vi "IPI_DrawLine.vi"(7 "Roi":dbl[](array[numeric]), 8 "error in (no error)":errorcluster, 9 "Distance Piex":string, 10 "Start Point":cluster{"X":dbl, "Y":dbl}, 11 "Image In":T1(plugin-control)) -> (0 "error out (no error)":errorcluster, 3 "Image Out":T1(plugin-control))   [LabVIEW 2015]
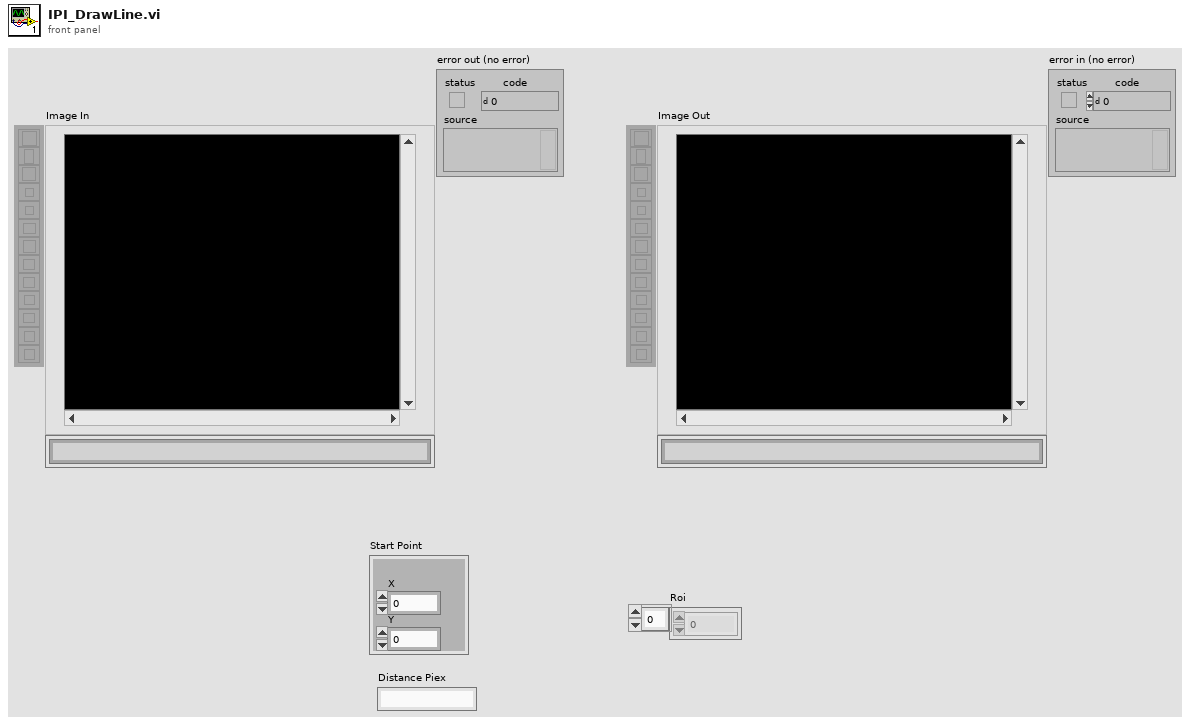
[diagram p1: front panel]
types:
  T1 = typedef "IMAQ Image.ctl" = refnum<image>
  T2 = cluster{"Left":i32, "Top":i32, "Right":i32, "Bottom":i32}
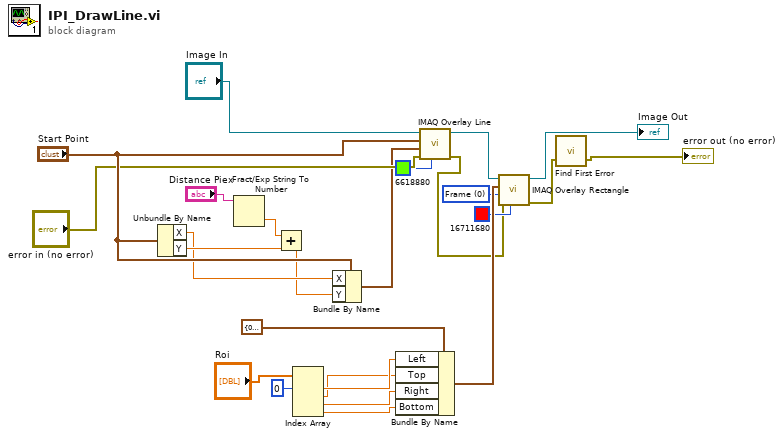
[diagram p0: block diagram]
diagram:
  w4 = u32 0 items=["Frame", "Fill", "Highlight"] ("Drawing Mode (Frame)")
  n1 = Unbundle By Name("Start Point") -> ("X"=w20:dbl, "Y"=w22:dbl)
  n2 = Fract/Exp String To Number(string="Distance Piex") -> (number=w23:dbl)  [unwired: 3 in, 1 out]
  n3 = Add(x=w23, y=w22) -> (x+y=w19:dbl)
  n4 = Index Array(array="Roi", index #1=0 ("索引")) -> (element #1=w10:dbl, element #2=w9:dbl, element #3=w8:dbl, element #4=w7:dbl)  [unwired: 3 in]
  n5 = Bundle By Name(cluster="Start Point", "X"=w20, "Y"=w19) -> (w17:cluster{"X":dbl, "Y":dbl})
  n6 = Bundle By Name(cluster=T2 {"Left"=0, "Top"=0, "Right"=0, "Bottom"=0} ("Rectangle"), "Left"=w10, "Top"=w9, "Right"=w8, "Bottom"=w7) -> (w5:T2)
  n7 = call "IMAQ Overlay Line"("Color"=u32 6618880, "error in (no error)"="error in (no error)", "End Point"=w17, "Start Point"="Start Point", "Image"="Image In") -> ("error out"=w2:errorcluster, "Image Out"=w14:T1)  [unwired: 5 in]
  n8 = call "IMAQ Overlay Rectangle"("Color"=u32 16711680, "error in (no error)"=w2, "Drawing Mode (Frame)"=w4, "Rectangle"=w5, "Image"=w14) -> ("error out"=w1:errorcluster, "Image Out"=→"Image Out":T1)  [unwired: 5 in]
  n9 = call <vilib>:"Find First Error.vi"("error in (no error)"=w1) -> ("error out"=→"error out (no error)":errorcluster)  [unwired: 3 in, 1 out]
